vi "Read Data reduction.vi"(8 "error in (no error)":errorcluster, 11 "Plot in":refnum<class "Plot.lvclass">) -> (0 "error out":errorcluster, 2 "Data reduction":T1={"Clip time"=FALSE, "Tiime 0"=0.0, "Time 1"=0.0, "Maximum data points"=1, "Decimation method"=enum."Min-Max"}, 3 "Plot out":refnum<class "Plot.lvclass">)   [LabVIEW 2019, in "Plot.lvclass"]
uses:
  Plot.lvclass
  NHMFL_Core/Libraries/File/Controls/Data reduction.ctl
  Plot.lvclass/Plot.ctl
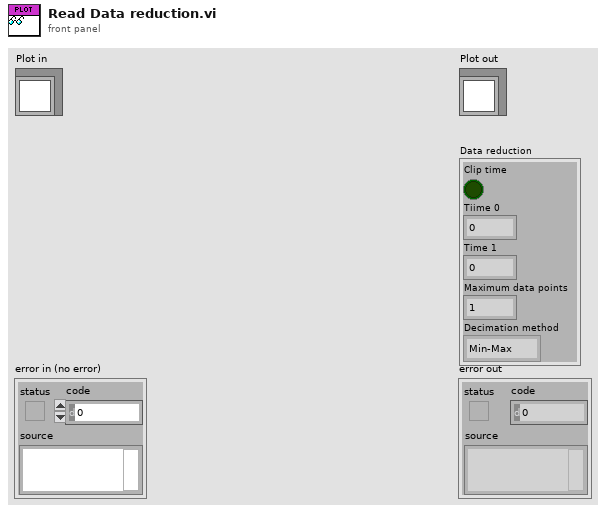
[diagram p1: front panel]
types:
  T1 = typedef "Data reduction.ctl" = cluster{"Clip time":bool, "Tiime 0":dbl, "Time 1":dbl, "Maximum data points":i32, "Decimation method":enum16{"coerce", "linear", "spline", "Min-Max", "Average"}}
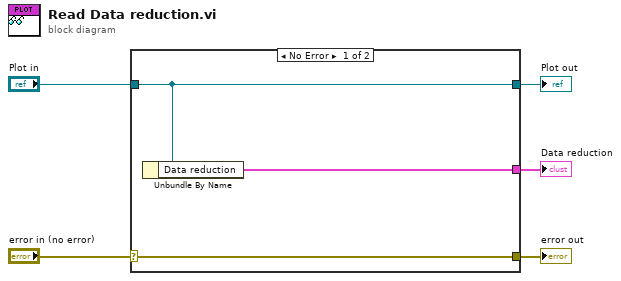
[diagram p0: block diagram]
diagram:
  n1 = case shown="No Error" "error in (no error)" {
    selector: "error in (no error)" -> [w8 w9]
    tunnel: [w8 w9] -> w4
    tunnel: [w7 w10] -> w2
    tunnel: "Plot in" -> [w7 w10]
    tunnel: [w6 _] -> w1
    frame No Error {
      n2 = Unbundle By Name(w7) -> ("Data reduction"=w6:T1)
    }
    frame Error {
    }
  }
  "error out" <- w4
  "Plot out" <- w2
  "Data reduction" <- w1
